vi "Update Tree Step Number.vi"(8 "New Step Number":i32, 9 "Old Step Number":i32, 11 "UI Data In":refnum<class "Settings UI.lvclass">) -> (0 "New Tag":string, 1 "Old Tag":string, 3 "UI Data Out":refnum<class "Settings UI.lvclass">)   [LabVIEW 2020, in "Output Sequencer.lvlib" / "Settings UI.lvclass"]
uses:
  Settings UI.lvclass
  Types/Tree Index Enum.ctl
  Settings UI.lvclass/Settings UI.ctl
  Globals/Global Tree Data.vi
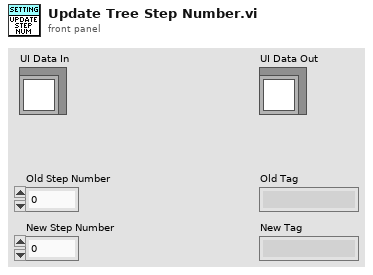
[diagram p1: front panel]
types:
  T1 = typedef "Output Sequencer.lvlib/Settings UI.lvclass/Tree Index Enum.ctl" = enum16{"General Settings", "Num Steps", "Num Analog", "Num Digital", "Show Confirmation", "Interp Priority", "Adv Timing", "Enable Conditions", "Seq Execution", "Reset Test Start", "Only When Test", "Delay After Test", "Start condition", "Re-triggering", "Stop condition", "Stop After Cycles", "Stop Values", "Default Values", "Default Analog", "Default Digital", "Steps", "Step #", "Description", "Precondition", "Duration", "Mode", "Delay Between Vals", "Analog Values", "Digital Values", "Postcondition", "On True", "On False"}
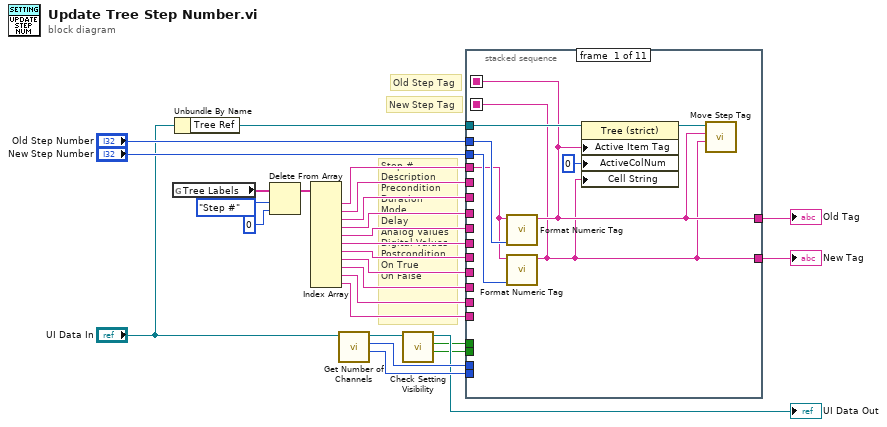
[diagram p0: block diagram]
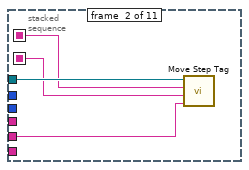
[diagram p2: hidden frame]
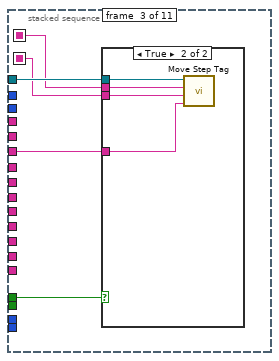
[diagram p3: hidden frame]
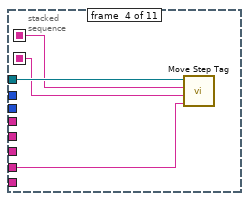
[diagram p5: hidden frame]
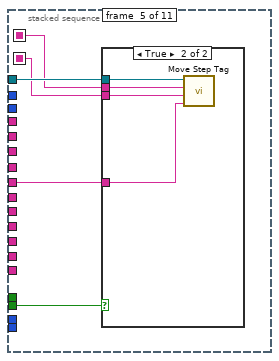
[diagram p6: hidden frame]
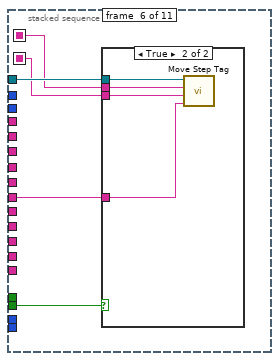
[diagram p8: hidden frame]
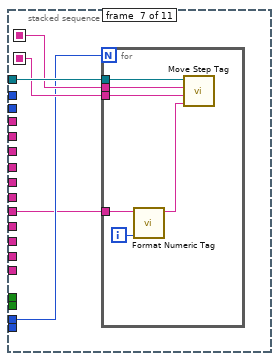
[diagram p10: hidden frame]
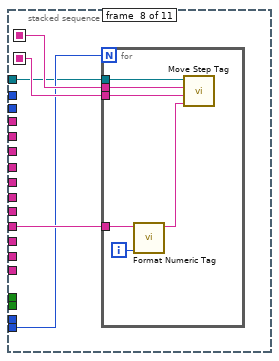
[diagram p11: hidden frame]
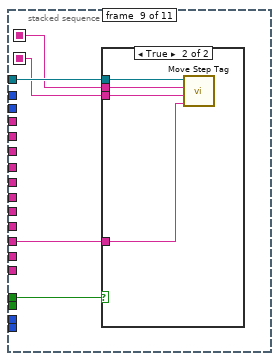
[diagram p12: hidden frame]
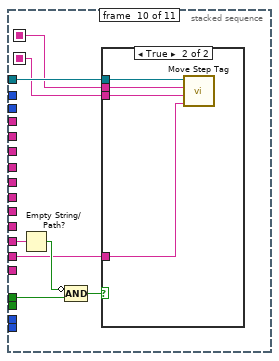
[diagram p14: hidden frame]
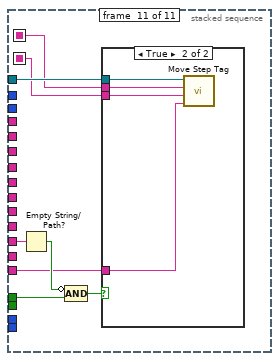
[diagram p16: hidden frame]
diagram:
  # "New Step Tag"
  # "Old Step Tag"
  # "Step #\nDescription\nPrecondition\nDuration\nMode\nDelay\nAnalog Values\nDigital Values\nPostcondition\nOn True\nOn False"
  n1 = global read "Global Tree Data.vi" "Tree Labels"() -> (w16:string[])
  n2 = Unbundle By Name("UI Data In") -> ("Tree Ref"=w1:refnum<vi>)
  n3 = Delete From Array(array=w16, length=Tree_Index_Enum."Step #" ("Tree Index Enum"), index=0) -> (array with subset deleted=w23:string[])  [unwired: 1 out]
  n4 = Index Array(array=w23) -> (element #1=w22:string, element #2=w18:string, element #3=w19:string, element #4=w20:string, element #5=w21:string, element #6=w17:string, element #7=w14:string, element #8=w11:string, element #9=w10:string, element #10=w9:string, element #11=w8:string)  [unwired: 11 in]
  n5 = call "Get Number of Channels.vi"("UI Data In"="UI Data In") -> ("Num of Digital Channels"=w12:i32, "Num of Analog Channels"=w13:i32, "UI Data out"=w3:refnum<class "Settings UI.lvclass">)  [unwired: 7 in, 1 out]
  n6 = call "Check Setting Visibility.vi"("UI Data in"=w3) -> ("Advanced timing visible"=w4:bool, "Conditional settings visible"=w5:bool, "UI Data out"=→"UI Data Out":refnum<class "Settings UI.lvclass">)  [unwired: 7 in, 1 out]
  n7 = stacked-sequence {
    seq-local: [w30 _ _ _ _ _ _ _ _ _ _] -> [_ w38 w40 w49 w54 w63 w74 w86 w95 w105 w117]
    seq-local: [w29 _ _ _ _ _ _ _ _ _ _] -> [_ w37 w41 w50 w53 w62 w73 w85 w94 w104 w116]
    tunnel: "Old Step Number" -> [w31 _ _ _ _ _ _ _ _ _ _]
    tunnel: w22 -> [w28 _ _ _ _ _ _ _ _ _ _]
    tunnel: w18 -> [_ w36 _ _ _ _ _ _ _ _ _]
    tunnel: w19 -> [_ _ w42 _ _ _ _ _ _ _ _]
    tunnel: w20 -> [_ _ _ w51 _ _ _ _ _ _ _]
    tunnel: w21 -> [_ _ _ _ w56 _ _ _ _ _ _]
    tunnel: w17 -> [_ _ _ _ _ w64 _ _ _ _ _]
    tunnel: "New Step Number" -> [w32 _ _ _ _ _ _ _ _ _ _]
    tunnel: w13 -> [_ _ _ _ _ _ w72 _ _ _ _]
    tunnel: w12 -> [_ _ _ _ _ _ _ w83 _ _ _]
    tunnel: w1 -> [w34 w39 w44 w52 w57 w66 w75 w82 w96 w106 w118]
    tunnel: [w29 _ _ _ _ _ _ _ _ _ _] -> w26
    tunnel: [w30 _ _ _ _ _ _ _ _ _ _] -> w15
    tunnel: w14 -> [_ _ _ _ _ _ w71 _ _ _ _]
    tunnel: w11 -> [_ _ _ _ _ _ _ w84 _ _ _]
    tunnel: w10 -> [_ _ _ _ _ _ _ _ w93 w109 w121]
    tunnel: w9 -> [_ _ _ _ _ _ _ _ _ w103 _]
    tunnel: w8 -> [_ _ _ _ _ _ _ _ _ _ w114]
    tunnel: w5 -> [_ _ w43 _ _ _ _ _ w97 w108 w120]
    tunnel: w4 -> [_ _ _ _ w55 w65 _ _ _ _ _]
    frame #0 {
      n8 = call "Format Numeric Tag.vi"("Number"=w31, "Tree label"=w28) -> ("Tag"=w30:string)  [unwired: 9 in]
      n9 = call "Format Numeric Tag.vi"("Number"=w32, "Tree label"=w28) -> ("Tag"=w29:string)  [unwired: 9 in]
      n10 = property class="Tree (strict)"(reference=w34, "Active Item Tag"=w30, "ActiveColNum"=0 ("Active Cell:Active Column Number"), "Cell String"=w29) -> (reference out=w33:refnum<vi>)  [unwired: 1 in, 1 out]
      n11 = call "Move Step Tag.vi"("New Step Tag"=w29, "Old Step Tag"=w30, "TreeControl in"=w33) -> ()  [unwired: 8 in, 1 out]
    }
    frame #1 {
      n12 = call "Move Step Tag.vi"("Child tag"=w36, "New Step Tag"=w37, "Old Step Tag"=w38, "TreeControl in"=w39) -> ()  [unwired: 7 in, 1 out]
    }
    frame #2 {
      n13 = case shown="True" w43 {
        tunnel: w44 -> [_ w48]
        tunnel: w42 -> [_ w45]
        tunnel: w41 -> [_ w46]
        tunnel: w40 -> [_ w47]
        frame False {
        }
        frame True {
          n14 = call "Move Step Tag.vi"("Child tag"=w45, "New Step Tag"=w46, "Old Step Tag"=w47, "TreeControl in"=w48) -> ()  [unwired: 7 in, 1 out]
        }
      }
    }
    frame #3 {
      n15 = call "Move Step Tag.vi"("Child tag"=w51, "New Step Tag"=w50, "Old Step Tag"=w49, "TreeControl in"=w52) -> ()  [unwired: 7 in, 1 out]
    }
    frame #4 {
      n16 = case shown="True" w55 {
        tunnel: w57 -> [_ w61]
        tunnel: w56 -> [_ w58]
        tunnel: w53 -> [_ w59]
        tunnel: w54 -> [_ w60]
        frame False {
        }
        frame True {
          n17 = call "Move Step Tag.vi"("Child tag"=w58, "New Step Tag"=w59, "Old Step Tag"=w60, "TreeControl in"=w61) -> ()  [unwired: 7 in, 1 out]
        }
      }
    }
    frame #5 {
      n18 = case shown="True" w65 {
        tunnel: w66 -> [_ w70]
        tunnel: w64 -> [_ w67]
        tunnel: w62 -> [_ w68]
        tunnel: w63 -> [_ w69]
        frame False {
        }
        frame True {
          n19 = call "Move Step Tag.vi"("Child tag"=w67, "New Step Tag"=w68, "Old Step Tag"=w69, "TreeControl in"=w70) -> ()  [unwired: 7 in, 1 out]
        }
      }
    }
    frame #6 {
      n20 = for {
        N: w72 -> [_]
        tunnel: w74 -> [w79]
        tunnel: w71 -> [w78]
        tunnel: w73 -> [w80]
        tunnel: w75 -> [w81]
        i -> [w77]
        n21 = call "Format Numeric Tag.vi"("Number"=w77, "Tree label"=w78) -> ("Tag"=w76:string)  [unwired: 9 in]
        n22 = call "Move Step Tag.vi"("Child tag"=w76, "New Step Tag"=w80, "Old Step Tag"=w79, "TreeControl in"=w81) -> ()  [unwired: 7 in, 1 out]
      }
    }
    frame #7 {
      n23 = for {
        N: w83 -> [_]
        tunnel: w86 -> [w90]
        tunnel: w84 -> [w87]
        tunnel: w85 -> [w91]
        tunnel: w82 -> [w92]
        i -> [w89]
        n24 = call "Format Numeric Tag.vi"("Number"=w89, "Tree label"=w87) -> ("Tag"=w88:string)  [unwired: 9 in]
        n25 = call "Move Step Tag.vi"("Child tag"=w88, "New Step Tag"=w91, "Old Step Tag"=w90, "TreeControl in"=w92) -> ()  [unwired: 7 in, 1 out]
      }
    }
    frame #8 {
      n26 = case shown="True" w97 {
        tunnel: w96 -> [_ w101]
        tunnel: w93 -> [_ w98]
        tunnel: w94 -> [_ w99]
        tunnel: w95 -> [_ w100]
        frame False {
        }
        frame True {
          n27 = call "Move Step Tag.vi"("Child tag"=w98, "New Step Tag"=w99, "Old Step Tag"=w100, "TreeControl in"=w101) -> ()  [unwired: 7 in, 1 out]
        }
      }
    }
    frame #9 {
      n28 = Empty String/Path?(string/path=w109) -> (empty?=w107:bool)
      n29 = Compound Arithmetic op=AND(invert w107, w108) -> (w102:bool)
      n30 = case shown="True" w102 {
        tunnel: w106 -> [_ w113]
        tunnel: w103 -> [_ w110]
        tunnel: w104 -> [_ w111]
        tunnel: w105 -> [_ w112]
        frame False {
        }
        frame True {
          n31 = call "Move Step Tag.vi"("Child tag"=w110, "New Step Tag"=w111, "Old Step Tag"=w112, "TreeControl in"=w113) -> ()  [unwired: 7 in, 1 out]
        }
      }
    }
    frame #10 {
      n32 = Empty String/Path?(string/path=w121) -> (empty?=w119:bool)
      n33 = Compound Arithmetic op=AND(invert w119, w120) -> (w115:bool)
      n34 = case shown="True" w115 {
        tunnel: w118 -> [_ w125]
        tunnel: w116 -> [_ w123]
        tunnel: w117 -> [_ w124]
        tunnel: w114 -> [_ w122]
        frame False {
        }
        frame True {
          n35 = call "Move Step Tag.vi"("Child tag"=w122, "New Step Tag"=w123, "Old Step Tag"=w124, "TreeControl in"=w125) -> ()  [unwired: 7 in, 1 out]
        }
      }
    }
  }
  "New Tag" <- w26
  "Old Tag" <- w15
